vi "Write Scope Resource.vi"(8 "error in (no error)":errorcluster, 9 "Simulated":bool, 10 "Scope Resource":refnum<visa-resource-name>, 11 "Unit_Test_Scope in":refnum<class "Unit_Test_Scope.lvclass">) -> (0 "error out":errorcluster, 3 "Unit_Test_Scope out":refnum<class "Unit_Test_Scope.lvclass">)   [LabVIEW 2020, in "Unit_Test_Scope.lvlib" / "Unit_Test_Scope.lvclass"]
uses:
  Unit_Test_Scope.lvclass
  Unit_Test_Scope.lvclass/Unit_Test_Scope.ctl
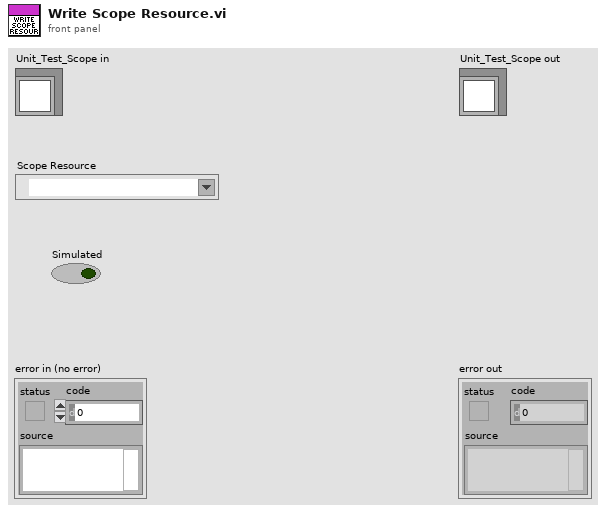
[diagram p1: front panel]
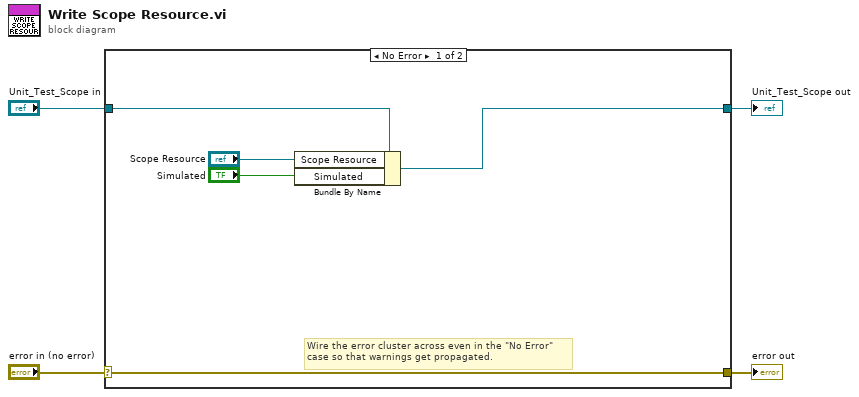
[diagram p0: block diagram]
diagram:
  n1 = case shown="No Error" "error in (no error)" {
    selector: "error in (no error)" -> [w9 w11]
    tunnel: [w9 w11] -> w3
    tunnel: [w5 w10] -> w1
    tunnel: "Unit_Test_Scope in" -> [w8 w10]
    frame No Error {
      # "Wire the error cluster across even in the \"No Error\"\ncase so that warnings get propagated."
      n2 = Bundle By Name(cluster=w8, "Scope Resource"="Scope Resource", "Simulated"="Simulated") -> (w5:refnum<class "Unit_Test_Scope.lvclass">)
    }
    frame Error {
    }
  }
  "error out" <- w3
  "Unit_Test_Scope out" <- w1
